vi "NXTDataPacketSnippet.vi"() -> ()   [LabVIEW 2010]
uses:
  <vilib>/NXT/Block Support/NXT_MessageMailbox.ctl
  <vilib>/NXT/Dual Mode Library/BT/BlueTooth_Write_String_toComputer.vi
panel:
  in  "BT Data Packet":T1
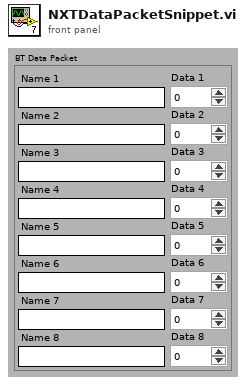
[diagram p1: front panel]
types:
  T1 = cluster{"Name 1":string, "Data 1":sgl, "Name 2":string, "Data 2":sgl, "Name 3":string, "Data 3":sgl, "Name 4":string, "Data 4":sgl, "Name 5":string, "Data 5":sgl, "Name 6":string, "Data 6":sgl, "Name 7":string, "Data 7":sgl, "Name 8":string, "Data 8":sgl}
  T2 = typedef "NXT_MessageMailbox.ctl" = u8
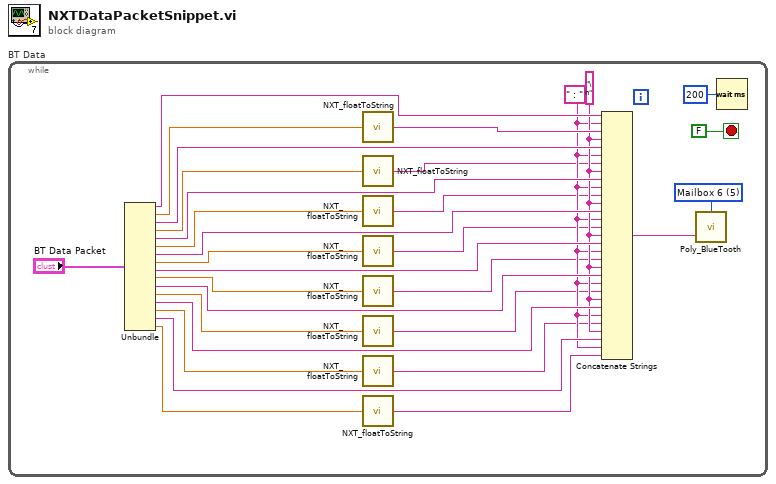
[diagram p0: block diagram]
diagram:
  n1 = while "BT Data" {
    stop <- FALSE stop-if-true
    w9 = "\n" ("string")
    w8 = " : " ("string")
    w29 = T2 5 items=["Mailbox 1", "Mailbox 2", "Mailbox 3", "Mailbox 4", "Mailbox 5", "Mailbox 6", "Mailbox 7", "Mailbox 8", "Mailbox 9", "Mailbox 10"] ("Mailbox")
    n2 = Unbundle("BT Data Packet") -> ("Name 1"=w19:string, "Data 1"=w27:sgl, "Name 2"=w17:string, "Data 2"=w26:sgl, "Name 3"=w16:string, "Data 3"=w25:sgl, "Name 4"=w15:string, "Data 4"=w24:sgl, "Name 5"=w14:string, "Data 5"=w23:sgl, "Name 6"=w13:string, "Data 6"=w22:sgl, "Name 7"=w12:string, "Data 7"=w21:sgl, "Name 8"=w11:string, "Data 8"=w20:sgl)
    n3 = call <vilib>:"NXT_floatToString.vi"("number"=w27) -> ("string"=w18:string)
    n4 = call <vilib>:"NXT_floatToString.vi"("number"=w26) -> ("string"=w7:string)
    n5 = call <vilib>:"NXT_floatToString.vi"("number"=w25) -> ("string"=w6:string)
    n6 = call <vilib>:"NXT_floatToString.vi"("number"=w24) -> ("string"=w5:string)
    n7 = call <vilib>:"NXT_floatToString.vi"("number"=w23) -> ("string"=w4:string)
    n8 = call <vilib>:"NXT_floatToString.vi"("number"=w22) -> ("string"=w3:string)
    n9 = call <vilib>:"NXT_floatToString.vi"("number"=w21) -> ("string"=w2:string)
    n10 = call <vilib>:"NXT_floatToString.vi"("number"=w20) -> ("string"=w10:string)
    n11 = Concatenate Strings(w19, w8, w18, w9, w17, w8, w7, w9, w16, w8, w6, w9, w15, w8, w5, w9, w14, w8, w4, w9, w13, w8, w3, w9, w12, w8, w2, w9, w11, w8, w10) -> (w1:string)
    n12 = call-poly <vilib>:"Poly_BlueTooth.vi"("Message in"=w1, "Mailbox"=w29) -> ()  [unwired: 2 in, 1 out]
    n13 = Wait (ms)(milliseconds to wait=u32 200) -> ()  [unwired: 1 out]
  }
